vi "Teleop.vi"(10 "Match Info":T1={"Autonomous Elapsed Seconds"=0.0, "TeleOp Elapsed Seconds"=0.0, "Disabled Elapsed Seconds"=0.0, "Visited Autonomous"=FALSE, "Visited TeleOp"=FALSE, "Visited Disabled"=FALSE, "Autonomous Settings"={"Autonomous Style"=enum."Independent", "VI Refnum"=refnum}}, 11 "Call Context":T2) -> ()   [LabVIEW 2019]
doc: "This VI is called for each TeleOp packet received from the DS where the robot is not disabled. It is often used to read from the joysticks and update I/O or to update setpoints for timed control loops. It should complete and return within 20 milliseconds or it may miss DS packets."
uses:
  <vilib>/Rock Robotics/WPI/DriverStation/WPI_DriverStationDerivedRobotMode.ctl
  <vilib>/Rock Robotics/WPI/DriverStation/WPI_DriverStationMatch Info.ctl
  <vilib>/Rock Robotics/WPI/Solenoid/WPI_SolenoidValue.ctl
  <vilib>/Rock Robotics/WPI/ThirdParty/Phoenix-LabVIEW/Motor Controller/Controls/CTRE_Phoenix_MotorControl_ControlMode.ctl
  <vilib>/Rock Robotics/WPI/ThirdParty/REV Robotics/SPARK MAX/Typedef/Spark MAX Control Type.ctl
  f70f45e1-7626-4a9c-a34c-83f61dc48ac5.vi
  <vilib>/Rock Robotics/WPI/Utilities/WPI_GetSetVariantRefNum.vi
  <vilib>/Rock Robotics/Network Tables/NT Write Boolean Array.vi
  <vilib>/Rock Robotics/Network Tables/NT Write Numeric Array.vi
  <vilib>/Rock Robotics/WPI/Solenoid/WPI_SolenoidSetEnum.vi
  <vilib>/Rock Robotics/Network Tables/NT Write Boolean.vi
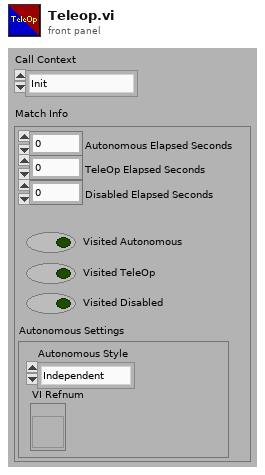
[diagram p1: front panel]
types:
  T1 = typedef "WPI_DriverStationMatch Info.ctl" = cluster{"Autonomous Elapsed Seconds":dbl, "TeleOp Elapsed Seconds":dbl, "Disabled Elapsed Seconds":dbl, "Visited Autonomous":bool, "Visited TeleOp":bool, "Visited Disabled":bool, "Autonomous Settings":cluster{"Autonomous Style":enum16{"Iterative", "Independent"}, "VI Refnum":refnum<vi>}}
  T2 = typedef "WPI_DriverStationDerivedRobotMode.ctl" = enum16{"Init", "Execute", "Stop"}
  T3 = typedef "CTRE_Phoenix_MotorControl_ControlMode.ctl" = u16
  T4 = typedef "WPI_SolenoidValue.ctl" = enum16{"Off", "On", "Forward", "Reverse"}
  T5 = typedef "WPI_JoystickDevRef.ctl" = cluster{"Device":T6}
  T6 = typedef "WPI_JoystickDeviceEnum.ctl" = enum16{"USB 0", "USB 1", "USB 2", "USB 3", "USB 4", "USB 5"}
  T7 = typedef "WPI_RobotDriveDevRef.ctl" = cluster{"DevStatus":errorcluster, "Motors[]":T8[], "Square Inputs":bool, "Max Output":dbl}
  T8 = typedef "WPI_MotorControlDeviceRef.ctl" = cluster{"DeviceStatus":errorcluster, "Type":T9, "PWM":cluster{"PWM Channel":T10, "DeadBand":T11}, "CAN":cluster{"Device Number":u8, "SetOutput VI Ref":variant, "GetOutput VI Ref":variant, "Enable VI Ref":variant, "Disable VI Ref":variant, "Data":variant}, "Invert":bool, "DIO PWM":cluster{"PWM \"Enable\" Channel":T10, "DIOChannel":T12, "PWM Rate":dbl}}
  T9 = typedef "WPI_MotorControlType.ctl" = enum16{"PWM", "CAN", "DIO PWM"}
  T10 = typedef "FPGA_DIOPWMChannel.ctl" = enum8{"PWM 0", "PWM 1", "PWM 2", "PWM 3", "PWM 4", "PWM 5", "PWM 6", "PWM 7", "PWM 8", "PWM 9", "PWM MXP 0", "PWM MXP 1", "PWM MXP 2", "PWM MXP 3", "PWM MXP 4", "PWM MXP 5", "PWM MXP 6", "PWM MXP 7", "PWM MXP 8", "PWM MXP 9", "Invalid"}
  T11 = typedef "WPI_PWMDeadband.ctl" = cluster{"Name":string, "maxPositivePwm":i32, "minPositivePwm":i32, "centerPwm":i32, "maxNegativePwm":i32, "minNegativePwm":i32, "angularRange":u16}
  T12 = typedef "FPGA_DIOChannel.ctl" = enum8{"DIO 0", "DIO 1", "DIO 2", "DIO 3", "DIO 4", "DIO 5", "DIO 6", "DIO 7", "DIO 8", "DIO 9", "DIO MXP 0", "DIO MXP 1", "DIO MXP 2", "DIO MXP 3", "DIO MXP 4", "DIO MXP 5", "DIO MXP 6", "DIO MXP 7", "DIO MXP 8", "DIO MXP 9", "DIO MXP 10", "DIO MXP 11", "DIO MXP 12", "DIO MXP 13", "DIO MXP 14", "DIO MXP 15", "SPI Port CS1", "SPI Port CS2", "SPI Port CS3", "SPI Port MISO", "SPI Port MOSI", "Invalid"}
  T13 = typedef "WPI_SolenoidDevRef.ctl" = cluster{"DevStatus":errorcluster, "Pneumatics Control Module":u8, "Forward Solenoid Channel":T14, "Reverse Solenoid Channel":T14}
  T14 = typedef "WPI_SolenoidChannel.ctl" = enum8{"Solenoid 0", "Solenoid 1", "Solenoid 2", "Solenoid 3", "Solenoid 4", "Solenoid 5", "Solenoid 6", "Solenoid 7", "Invalid"}
  T15 = typedef "WPI_DigitalInputDevRef.ctl" = cluster{"DevStatus":errorcluster, "DIO Channel":T12}
  T16 = typedef "Spark MAX Control Type.ctl" = enum16{"Percent VBus", "Voltage", "Velocity", "Position", "Smart Motion", "Current", "Smart Velocity"}
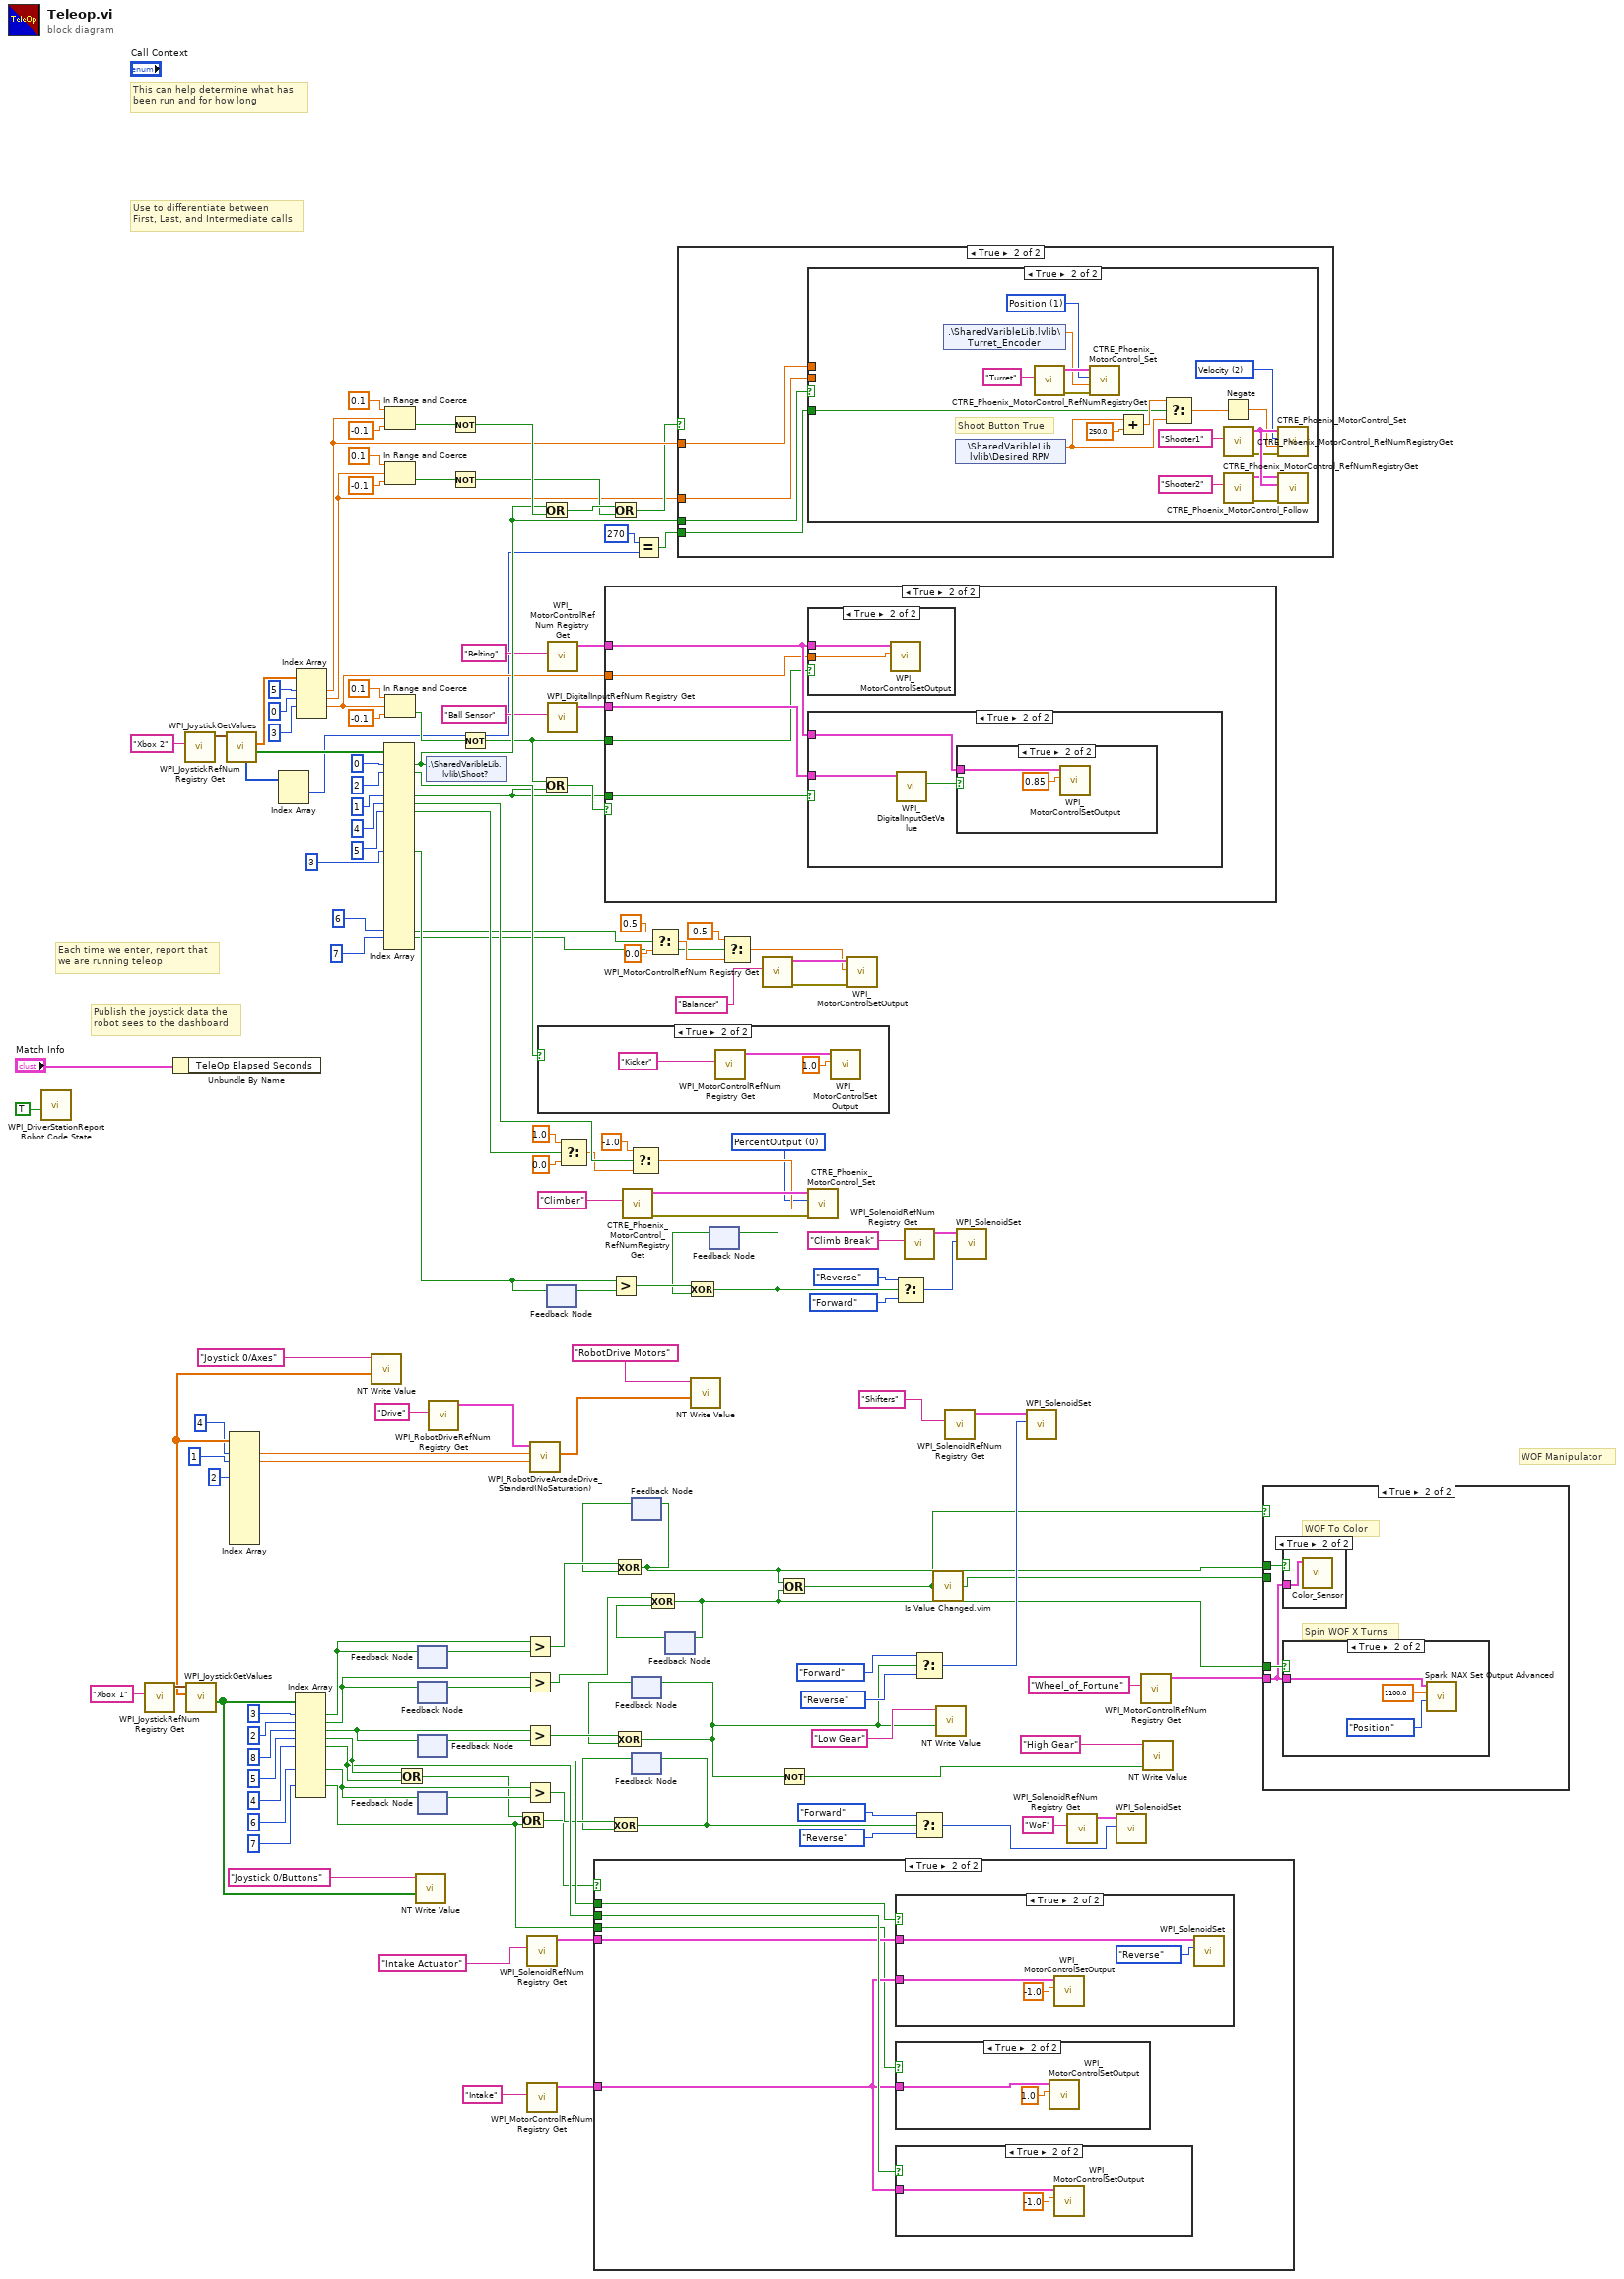
[diagram p0: block diagram]
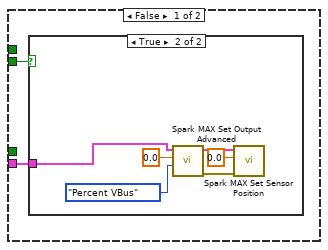
[diagram p2: hidden frame]
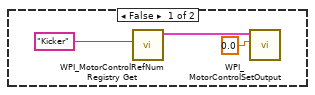
[diagram p6: hidden frame]
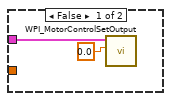
[diagram p7: hidden frame]
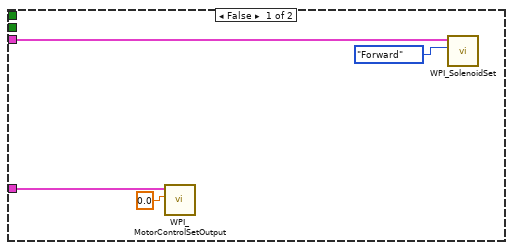
[diagram p11: hidden frame]
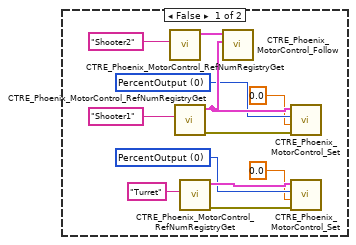
[diagram p15: hidden frame]
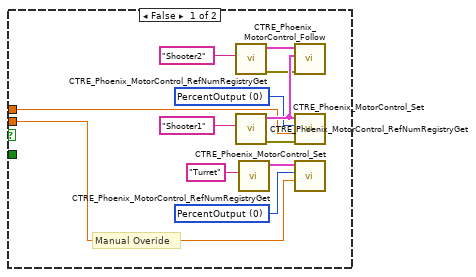
[diagram p16: hidden frame]
diagram:
  w23 = T3 0 items=["PercentOutput"=0, "Position"=1, "Velocity"=2, "Current"=3, "Follower"=5, "MotionProfile"=6, "MotionMagic"=7, "MotionProfileArc"=10, "Disabled"=15] ("Control Mode")
  # "WOF Manipulator"
  # "Publish the joystick data the\nrobot sees to the dashboard"
  # "Each time we enter, report that\nwe are running teleop"
  # "Use to differentiate between\nFirst, Last, and Intermediate calls"
  # "This can help determine what has\nbeen run and for how long"
  n1 = call <vilib>:"WPI_DriverStationReport Robot Code State.vi"("TeleOp"=TRUE ("Autonomous")) -> ()  [unwired: 10 in, 1 out]
  n2 = call <vilib>:"WPI_JoystickRefNum Registry Get.vi"("refnum name"="Xbox 1") -> ("JoystickDevRef"=w143:T5)  [unwired: 1 in, 9 out]
  n3 = Unbundle By Name("Match Info") -> ()  [unwired: 1 out]
  n4 = call <vilib>:"WPI_JoystickRefNum Registry Get.vi"("refnum name"="Xbox 2") -> ("JoystickDevRef"=w118:T5)  [unwired: 1 in, 9 out]
  n5 = call <vilib>:"WPI_JoystickGetValues.vi"("JoystickDevRef"=w143) -> ("Buttons"=w136:bool[], "Axes"=w139:dbl[])  [unwired: 6 in, 3 out]
  n6 = call <vilib>:"WPI_JoystickGetValues.vi"("JoystickDevRef"=w118) -> ("Buttons"=w116:bool[], "Axes"=w117:dbl[], "POVs"=w18:i16[])  [unwired: 6 in, 2 out]
  n7 = Index Array(array=w139, index #1=4 ("index"), index #2=1 ("index"), index #4=2 ("index")) -> (element #1=w75:dbl, element #2=w76:dbl)  [unwired: 9 in, 10 out]
  n8 = Index Array(array=w18) -> (element #1=w17:i16)  [unwired: 2 in, 1 out]
  n9 = Index Array(array=w136, index #1=3 ("index"), index #2=2 ("index"), index #3=8 ("index"), index #4=5 ("index"), index #5=4 ("index"), index #8=6 ("index"), index #10=7 ("index")) -> (element #1=w132:bool, element #2=w131:bool, element #3=w120:bool, element #4=w74:bool, element #5=w72:bool, element #8=w62:bool, element #10=w33:bool)  [unwired: 4 in, 4 out]
  n10 = Index Array(array=w117, index #1=5 ("index"), index #2=0 ("index"), index #3=3 ("index")) -> (element #1=w106:dbl, element #2=w100:dbl, element #3=w51:dbl)  [unwired: 1 in, 1 out]
  n11 = call-poly <vilib>:"NT Write Value.vi"("Numeric Array"=w139, "Name"="Joystick 0/Axes") -> ()  [unwired: 9 in, 1 out]
  n12 = Index Array(array=w116, index #1=0 ("index"), index #2=2 ("index"), index #5=1 ("index"), index #6=4 ("index"), index #7=5 ("index"), index #12=3 ("index"), index #22=6 ("index"), index #23=7 ("index")) -> (element #1=w105:bool, element #2=w97:bool, element #5=w53:bool, element #6=w49:bool, element #7=w48:bool, element #12=w37:bool, element #22=w4:bool, element #23=w3:bool)  [unwired: 16 in, 16 out]
  n13 = In Range and Coerce(upper limit=0.1, x=w106, lower limit=-0.1) -> (In Range?=w114:bool)  [unwired: 1 out]
  n14 = In Range and Coerce(upper limit=0.1, x=w100, lower limit=-0.1) -> (In Range?=w104:bool)  [unwired: 1 out]
  n15 = In Range and Coerce(upper limit=0.1, x=w51, lower limit=-0.1) -> (In Range?=w55:bool)  [unwired: 1 out]
  n16 = Or(x=w74, y=w72) -> (x .or. y?=w32:bool)
  n17 = call-poly <vilib>:"NT Write Value.vi"("Boolean Array"=w136, "Name"="Joystick 0/Buttons") -> ()  [unwired: 9 in, 1 out]
  n18 = feedback #1() -> (w94:bool)  [unwired: 1 in]
  n19 = feedback-in #1(w132) -> ()
  n20 = feedback #2() -> (w91:bool)  [unwired: 1 in]
  n21 = feedback-in #2(w131) -> ()
  n22 = feedback #3() -> (w130:bool)  [unwired: 1 in]
  n23 = feedback-in #3(w120) -> ()
  n24 = feedback #4() -> (w66:bool)  [unwired: 1 in]
  n25 = feedback-in #4(w62) -> ()
  n26 = shared-variable ".\\SharedVaribleLib.lvlib\\Shoot?"(w105) -> ()  [unwired: 1 in, 1 out]
  n27 = call <vilib>:"WPI_RobotDriveRefNum Registry Get.vi"("refnum name"="Drive") -> ("RobotDriveDevRef"=w60:T7)  [unwired: 1 in, 9 out]
  n28 = Not(x=w114) -> (.not. x?=w113:bool)
  n29 = Not(x=w104) -> (.not. x?=w102:bool)
  n30 = Not(x=w55) -> (.not. x?=w52:bool)
  n31 = Or(x=w32, y=w33) -> (x .or. y?=w31:bool)
  n32 = Greater?(x=w132, y=w94) -> (0:w93:bool)
  n33 = Greater?(x=w131, y=w91) -> (0:w90:bool)
  n34 = Greater?(x=w120, y=w130) -> (0:w129:bool)
  n35 = Greater?(x=w62, y=w66) -> (0:w65:bool)
  n36 = call <vilib>:"WPI_SolenoidRefNum Registry Get.vi"("refnum name"="Intake Actuator") -> ("SolenoidDevRef"=w81:T13)  [unwired: 9 in, 1 out]
  n37 = call <vilib>:"WPI_MotorControlRefNum Registry Get.vi"("refnum name"="Intake") -> ("MotorControlDevRef"=w83:T8)  [unwired: 9 in, 1 out]
  n38 = call <vilib>:"WPI_RobotDriveArcadeDrive_Standard(NoSaturation).vi"("Y axis value"=w76, "X axis value"=w75, "RobotDriveDevRef"=w60) -> ("Motor Values"=w59:dbl[])  [unwired: 1 in, 7 out]
  n39 = case shown="True" w97 {
    frame False {
      n40 = call <vilib>:"WPI_MotorControlRefNum Registry Get.vi"("refnum name"="Kicker") -> ("MotorControlDevRef"=w148:T8)  [unwired: 9 in, 1 out]
      n41 = call <vilib>:"WPI_MotorControlSetOutput.vi"("Output"=0.0, "MotorControlDevRef"=w148) -> ()  [unwired: 7 in, 3 out]
    }
    frame True {
      n42 = call <vilib>:"WPI_MotorControlRefNum Registry Get.vi"("refnum name"="Kicker") -> ("MotorControlDevRef"=w151:T8)  [unwired: 9 in, 1 out]
      n43 = call <vilib>:"WPI_MotorControlSetOutput.vi"("Output"=1.0, "MotorControlDevRef"=w151) -> ()  [unwired: 7 in, 3 out]
    }
  }
  n44 = Or(x=w105, y=w113) -> (x .or. y?=w103:bool)
  n45 = Or(x=w52, y=w53) -> (x .or. y?=w54:bool)
  n46 = feedback #5() -> (w36:bool)  [unwired: 1 in]
  n47 = feedback-in #5(w37) -> ()
  n48 = call <vilib>:"WPI_MotorControlRefNum Registry Get.vi"("refnum name"="Belting") -> ("MotorControlDevRef"=w79:T8)  [unwired: 9 in, 1 out]
  n49 = call <vilib>:"WPI_DigitalInputRefNum Registry Get.vi"("refnum name"="Ball Sensor") -> ("DigitalInputDevRef"=w77:T15)  [unwired: 9 in, 1 out]
  n50 = Select(t=1.0, s=w48, f=0.0) -> (s? t:f=w26:dbl)
  n51 = case shown="True" w31 {
    tunnel: w74 -> [_ w160]
    tunnel: w72 -> [_ w159]
    tunnel: w83 -> [w153 w157]
    tunnel: w81 -> [w152 w158]
    tunnel: w33 -> [_ w156]
    frame False {
      n52 = call <vilib>:"WPI_MotorControlSetOutput.vi"("Output"=0.0, "MotorControlDevRef"=w153) -> ()  [unwired: 7 in, 3 out]
      n53 = call-poly <vilib>:"WPI_SolenoidSet.vi"("Value"=WPI_SolenoidValue."Forward", "SolenoidDevRef"=w152) -> ()  [unwired: 8 in, 2 out]
    }
    frame True {
      n54 = case shown="True" w160 {
        tunnel: w157 -> [_ w167]
        tunnel: w158 -> [_ w166]
        frame False {
        }
        frame True {
          n55 = call <vilib>:"WPI_MotorControlSetOutput.vi"("Output"=-1.0, "MotorControlDevRef"=w167) -> ()  [unwired: 7 in, 3 out]
          n56 = call-poly <vilib>:"WPI_SolenoidSet.vi"("Value"=WPI_SolenoidValue."Reverse", "SolenoidDevRef"=w166) -> ()  [unwired: 8 in, 2 out]
        }
      }
      n57 = case shown="True" w156 {
        tunnel: w157 -> [_ w161]
        frame False {
        }
        frame True {
          n58 = call <vilib>:"WPI_MotorControlSetOutput.vi"("Output"=1.0, "MotorControlDevRef"=w161) -> ()  [unwired: 7 in, 3 out]
        }
      }
      n59 = case shown="True" w159 {
        tunnel: w157 -> [_ w163]
        frame False {
        }
        frame True {
          n60 = call <vilib>:"WPI_MotorControlSetOutput.vi"("Output"=-1.0, "MotorControlDevRef"=w163) -> ()  [unwired: 7 in, 3 out]
        }
      }
    }
  }
  n61 = case shown="True" w54 {
    tunnel: w79 -> [w169 w175]
    tunnel: w77 -> [_ w174]
    tunnel: w53 -> [_ w173]
    tunnel: w52 -> [_ w172]
    tunnel: w51 -> [_ w171]
    frame False {
      n62 = call <vilib>:"WPI_MotorControlSetOutput.vi"("Output"=0.0, "MotorControlDevRef"=w169) -> ()  [unwired: 7 in, 3 out]
    }
    frame True {
      n63 = case shown="True" w172 {
        tunnel: w175 -> [_ w177]
        tunnel: w171 -> [_ w176]
        frame False {
        }
        frame True {
          n64 = call <vilib>:"WPI_MotorControlSetOutput.vi"("Output"=w176, "MotorControlDevRef"=w177) -> ()  [unwired: 7 in, 3 out]
        }
      }
      n65 = case shown="True" w173 {
        tunnel: w175 -> [_ w179]
        tunnel: w174 -> [_ w178]
        frame False {
        }
        frame True {
          n66 = call <vilib>:"WPI_DigitalInputGetValue.vi"("DigitalInputDevRef"=w178) -> ("Value"=w180:bool)  [unwired: 8 in, 2 out]
          n67 = case shown="True" w180 {
            tunnel: w179 -> [_ w181]
            frame False {
            }
            frame True {
              n68 = call <vilib>:"WPI_MotorControlSetOutput.vi"("Output"=0.85, "MotorControlDevRef"=w181) -> ()  [unwired: 7 in, 3 out]
            }
          }
        }
      }
    }
  }
  n69 = Or(x=w103, y=w102) -> (x .or. y?=w101:bool)
  n70 = Greater?(x=w37, y=w36) -> (0:w40:bool)
  n71 = call <vilib>:"CTRE_Phoenix_MotorControl_RefNumRegistryGet.vi"("refnum name"="Climber") -> ("error out"=w29:errorcluster, "PhoenixMotorControlDevRef"=w30:T8)  [unwired: 9 in]
  n72 = Select(t=-1.0, s=w49, f=w26) -> (s? t:f=w24:dbl)
  n73 = feedback #6() -> (w92:bool)  [unwired: 1 in]
  n74 = Exclusive Or(1:w92, 2:w93) -> (0:w88:bool)
  n75 = feedback-in #6(w88) -> ()
  n76 = feedback #7() -> (w128:bool)  [unwired: 1 in]
  n77 = Exclusive Or(1:w128, 2:w129) -> (0:w20:bool)
  n78 = feedback-in #7(w20) -> ()
  n79 = feedback #8() -> (w64:bool)  [unwired: 1 in]
  n80 = Exclusive Or(1:w64, 2:w65) -> (0:w63:bool)
  n81 = feedback-in #8(w63) -> ()
  n82 = Equal?(x=i16 270, y=w17) -> (x = y?=w19:bool)
  n83 = Select(t=0.5, s=w4, f=0.0) -> (s? t:f=w9:dbl)
  n84 = feedback #9() -> (w89:bool)  [unwired: 1 in]
  n85 = Exclusive Or(1:w89, 2:w90) -> (0:w87:bool)
  n86 = feedback-in #9(w87) -> ()
  n87 = case shown="True" w101 {
    tunnel: w106 -> [_ w198]
    tunnel: w105 -> [_ w197]
    tunnel: w100 -> [_ w196]
    tunnel: w19 -> [_ w195]
    frame False {
      w184 = T3 0 items=["PercentOutput"=0, "Position"=1, "Velocity"=2, "Current"=3, "Follower"=5, "MotionProfile"=6, "MotionMagic"=7, "MotionProfileArc"=10, "Disabled"=15] ("Control Mode")
      w191 = T3 0 items=["PercentOutput"=0, "Position"=1, "Velocity"=2, "Current"=3, "Follower"=5, "MotionProfile"=6, "MotionMagic"=7, "MotionProfileArc"=10, "Disabled"=15] ("Control Mode")
      n88 = call <vilib>:"CTRE_Phoenix_MotorControl_RefNumRegistryGet.vi"("refnum name"="Shooter2") -> ("PhoenixMotorControlDevRef"=w192:T8)  [unwired: 9 in, 1 out]
      n89 = call <vilib>:"CTRE_Phoenix_MotorControl_RefNumRegistryGet.vi"("refnum name"="Shooter1") -> ("error out"=w190:errorcluster, "PhoenixMotorControlDevRef"=w194:T8)  [unwired: 9 in]
      n90 = call <vilib>:"CTRE_Phoenix_MotorControl_RefNumRegistryGet.vi"("refnum name"="Turret") -> ("error out"=w186:errorcluster, "PhoenixMotorControlDevRef"=w187:T8)  [unwired: 9 in]
      n91 = call <vilib>:"CTRE_Phoenix_MotorControl_Follow.vi"("Master Controller to Follow"=w194, "PhoenixMotorControlDevRef"=w192) -> ()  [unwired: 8 in, 2 out]
      n92 = call <vilib>:"CTRE_Phoenix_MotorControl_Set.vi"("error in (no error)"=w190, "Output"=0.0 ("upper limit"), "Control Mode"=w191, "PhoenixMotorControlDevRef"=w194) -> ()  [unwired: 6 in, 2 out]
      n93 = call <vilib>:"CTRE_Phoenix_MotorControl_Set.vi"("error in (no error)"=w186, "Output"=0.0, "Control Mode"=w184, "PhoenixMotorControlDevRef"=w187) -> ()  [unwired: 6 in, 2 out]
    }
    frame True {
      n94 = case shown="True" w197 {
        tunnel: w198 -> [w203 _]
        tunnel: w196 -> [w199 _]
        tunnel: w195 -> [_ w216]
        frame False {
          w200 = T3 0 items=["PercentOutput"=0, "Position"=1, "Velocity"=2, "Current"=3, "Follower"=5, "MotionProfile"=6, "MotionMagic"=7, "MotionProfileArc"=10, "Disabled"=15] ("Control Mode")
          w206 = T3 0 items=["PercentOutput"=0, "Position"=1, "Velocity"=2, "Current"=3, "Follower"=5, "MotionProfile"=6, "MotionMagic"=7, "MotionProfileArc"=10, "Disabled"=15] ("Control Mode")
          # "Manual Overide"
          n95 = call <vilib>:"CTRE_Phoenix_MotorControl_RefNumRegistryGet.vi"("refnum name"="Shooter2") -> ("error out"=w208:errorcluster, "PhoenixMotorControlDevRef"=w207:T8)  [unwired: 9 in]
          n96 = call <vilib>:"CTRE_Phoenix_MotorControl_RefNumRegistryGet.vi"("refnum name"="Shooter1") -> ("error out"=w205:errorcluster, "PhoenixMotorControlDevRef"=w210:T8)  [unwired: 9 in]
          n97 = call <vilib>:"CTRE_Phoenix_MotorControl_RefNumRegistryGet.vi"("refnum name"="Turret") -> ("PhoenixMotorControlDevRef"=w202:T8)  [unwired: 9 in, 1 out]
          n98 = call <vilib>:"CTRE_Phoenix_MotorControl_Follow.vi"("error in (no error)"=w208, "Master Controller to Follow"=w210, "PhoenixMotorControlDevRef"=w207) -> ()  [unwired: 7 in, 2 out]
          n99 = call <vilib>:"CTRE_Phoenix_MotorControl_Set.vi"("error in (no error)"=w205, "Output"=w203, "Control Mode"=w206, "PhoenixMotorControlDevRef"=w210) -> ()  [unwired: 6 in, 2 out]
          n100 = call <vilib>:"CTRE_Phoenix_MotorControl_Set.vi"("Output"=w199, "Control Mode"=w200, "PhoenixMotorControlDevRef"=w202) -> ()  [unwired: 7 in, 2 out]
        }
        frame True {
          w212 = T3 1 items=["PercentOutput"=0, "Position"=1, "Velocity"=2, "Current"=3, "Follower"=5, "MotionProfile"=6, "MotionMagic"=7, "MotionProfileArc"=10, "Disabled"=15] ("Control Mode")
          w224 = T3 2 items=["PercentOutput"=0, "Position"=1, "Velocity"=2, "Current"=3, "Follower"=5, "MotionProfile"=6, "MotionMagic"=7, "MotionProfileArc"=10, "Disabled"=15] ("Control Mode")
          # "Shoot Button True"
          n101 = shared-variable ".\\SharedVaribleLib.lvlib\\Turret_Encoder"() -> (w211:dbl)  [unwired: 1 in, 1 out]
          n102 = shared-variable ".\\SharedVaribleLib.lvlib\\Desired RPM"() -> (w217:dbl)  [unwired: 1 in, 1 out]
          n103 = call <vilib>:"CTRE_Phoenix_MotorControl_RefNumRegistryGet.vi"("refnum name"="Turret") -> ("error out"=w214:errorcluster, "PhoenixMotorControlDevRef"=w215:T8)  [unwired: 9 in]
          n104 = call <vilib>:"CTRE_Phoenix_MotorControl_Set.vi"("error in (no error)"=w214, "Output"=w211, "Control Mode"=w212, "PhoenixMotorControlDevRef"=w215) -> ()  [unwired: 6 in, 2 out]
          n105 = Add(x=w217, y=250.0) -> (x+y=w219:dbl)
          n106 = Select(t=w219, s=w216, f=w217) -> (s? t:f=w220:dbl)
          n107 = Negate(x=w220) -> (-x=w222:dbl)
          n108 = call <vilib>:"CTRE_Phoenix_MotorControl_RefNumRegistryGet.vi"("refnum name"="Shooter1") -> ("error out"=w223:errorcluster, "PhoenixMotorControlDevRef"=w228:T8)  [unwired: 9 in]
          n109 = call <vilib>:"CTRE_Phoenix_MotorControl_RefNumRegistryGet.vi"("refnum name"="Shooter2") -> ("error out"=w226:errorcluster, "PhoenixMotorControlDevRef"=w225:T8)  [unwired: 9 in]
          n110 = call <vilib>:"CTRE_Phoenix_MotorControl_Set.vi"("error in (no error)"=w223, "Output"=w222, "Control Mode"=w224, "PhoenixMotorControlDevRef"=w228) -> ()  [unwired: 6 in, 2 out]
          n111 = call <vilib>:"CTRE_Phoenix_MotorControl_Follow.vi"("error in (no error)"=w226, "Master Controller to Follow"=w228, "PhoenixMotorControlDevRef"=w225) -> ()  [unwired: 7 in, 2 out]
        }
      }
    }
  }
  n112 = call-poly <vilib>:"NT Write Value.vi"("Numeric Array"=w59, "Name"="RobotDrive Motors") -> ()  [unwired: 9 in, 1 out]
  n113 = feedback #10() -> (w39:bool)  [unwired: 1 in]
  n114 = Exclusive Or(1:w39, 2:w40) -> (0:w38:bool)
  n115 = feedback-in #10(w38) -> ()
  n116 = Select(t=-0.5, s=w3, f=w9) -> (s? t:f=w7:dbl)
  n117 = call <vilib>:"WPI_MotorControlRefNum Registry Get.vi"("refnum name"="Balancer") -> ("error out"=w12:errorcluster, "MotorControlDevRef"=w11:T8)  [unwired: 9 in]
  n118 = Or(x=w88, y=w87) -> (x .or. y?=w86:bool)
  n119 = Not(x=w20) -> (.not. x?=w21:bool)
  n120 = call <vilib>:"CTRE_Phoenix_MotorControl_Set.vi"("error in (no error)"=w29, "Output"=w24, "Control Mode"=w23, "PhoenixMotorControlDevRef"=w30) -> ()  [unwired: 6 in, 2 out]
  n121 = call <vilib>:"WPI_MotorControlSetOutput.vi"("error in (no error)"=w12, "Output"=w7, "MotorControlDevRef"=w11) -> ()  [unwired: 6 in, 3 out]
  n122 = Select(t=WPI_SolenoidValue."Reverse" ("Value"), s=w38, f=WPI_SolenoidValue."Forward" ("Value")) -> (s? t:f=w43:T4)
  n123 = call <vilib>:"WPI_SolenoidRefNum Registry Get.vi"("refnum name"="Climb Break") -> ("SolenoidDevRef"=w41:T13)  [unwired: 9 in, 1 out]
  n124 = Select(t=WPI_SolenoidValue."Forward" ("Value"), s=w20, f=WPI_SolenoidValue."Reverse" ("Value")) -> (s? t:f=w125:T4)
  n125 = Select(t=WPI_SolenoidValue."Forward" ("Value"), s=w63, f=WPI_SolenoidValue."Reverse" ("Value")) -> (s? t:f=w69:T4)
  n126 = call "Is Value Changed.vim"("value"=w86) -> ("changed or first call?"=w85:bool)
  n127 = call-poly <vilib>:"NT Write Value.vi"("Boolean"=w20, "Name"="Low Gear") -> ()  [unwired: 9 in, 1 out]
  n128 = call <vilib>:"WPI_SolenoidRefNum Registry Get.vi"("refnum name"="Shifters") -> ("SolenoidDevRef"=w123:T13)  [unwired: 9 in, 1 out]
  n129 = call-poly <vilib>:"WPI_SolenoidSet.vi"("Value"=w43, "SolenoidDevRef"=w41) -> ()  [unwired: 8 in, 2 out]
  n130 = call-poly <vilib>:"WPI_SolenoidSet.vi"("Value"=w125, "SolenoidDevRef"=w123) -> ()  [unwired: 8 in, 2 out]
  n131 = call <vilib>:"WPI_SolenoidRefNum Registry Get.vi"("refnum name"="WoF") -> ("SolenoidDevRef"=w67:T13)  [unwired: 9 in, 1 out]
  n132 = call-poly <vilib>:"WPI_SolenoidSet.vi"("Value"=w69, "SolenoidDevRef"=w67) -> ()  [unwired: 8 in, 2 out]
  n133 = call <vilib>:"WPI_MotorControlRefNum Registry Get.vi"("refnum name"="Wheel_of_Fortune") -> ("MotorControlDevRef"=w14:T8)  [unwired: 9 in, 1 out]
  n134 = call-poly <vilib>:"NT Write Value.vi"("Boolean"=w21, "Name"="High Gear") -> ()  [unwired: 9 in, 1 out]
  n135 = case shown="True" w86 {
    tunnel: w88 -> [_ w239]
    tunnel: w14 -> [w230 w237]
    tunnel: w87 -> [_ w238]
    tunnel: w85 -> [w229 _]
    frame False {
      n136 = case shown="True" w229 {
        tunnel: w230 -> [_ w234]
        frame False {
        }
        frame True {
          n137 = call <vilib>:"Spark MAX Set Output Advanced.vi"("Control Mode"=Spark_MAX_Control_Type."Percent VBus", "Setpoint"=0.0, "MotorControlDevRef"=w234) -> ("error out"=w233:errorcluster, "MotorControlDevRef"=w232:T8)  [unwired: 7 in]
          n138 = call <vilib>:"Spark MAX Set Sensor Position.vi"("error in"=w233, "Position"=0.0, "MotorControlDeviceRef"=w232) -> ()  [unwired: 7 in, 2 out]
        }
      }
    }
    frame True {
      # "WOF To Color"
      # "Spin WOF X Turns"
      n139 = case shown="True" w239 {
        tunnel: w237 -> [_ w243]
        frame False {
        }
        frame True {
          n140 = call "Color_Sensor.vi"("MotorControlDevRef"=w243) -> ()  [unwired: 11 in]
        }
      }
      n141 = case shown="True" w238 {
        tunnel: w237 -> [_ w242]
        frame False {
        }
        frame True {
          n142 = call <vilib>:"Spark MAX Set Output Advanced.vi"("Control Mode"=Spark_MAX_Control_Type."Position", "Setpoint"=1100.0, "MotorControlDevRef"=w242) -> ()  [unwired: 7 in, 2 out]
        }
      }
    }
  }
